vi "005 ascii.vi"() -> ()   [LabVIEW 2019]
panel:
  out "*(type *) &x":u8
  in  "Lletra":string
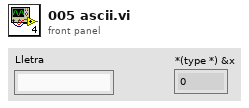
[diagram p1: front panel]
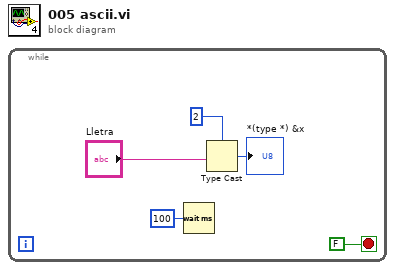
[diagram p0: block diagram]
diagram:
  n1 = while {
    stop <- FALSE stop-if-true
    n2 = Wait (ms)(milliseconds to wait=u32 100) -> ()  [unwired: 1 out]
    n3 = Type Cast(type=u8 2, x="Lletra") -> (*(type *) &x=→"*(type *) &x":u8)
  }
